vi "Waveform Input.vi"(8 "error in (no error)":errorcluster, 11 "Node Ptr":T1 format="%.0x") -> (0 "error out":errorcluster)   [LabVIEW 2019, in "FPGA Addon System Explorer.lvlib"]
uses:
  FPGA Addon System Explorer.lvlib
  <vilib>/NI VeriStand/Custom Device API/Custom Device Item Ref.ctl
  <vilib>/NI VeriStand/Custom Device API/Custom Device API.lvlib
panel:
  out "Original Name":string
  in  "Units":string
  in  "Header":cluster{"Section Name":string}={"Section Name"="Waveform Input Settings"}
  in  "Description":string
  in  "Name":string
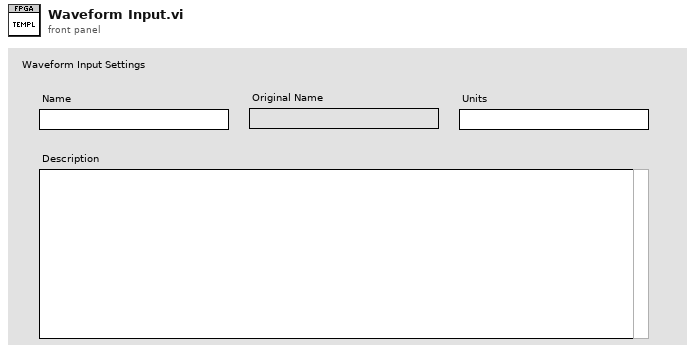
[diagram p1: front panel]
types:
  T1 = typedef "Custom Device API.lvlib/Custom Device Item Ref.ctl" = u64
  T2 = typedef "Custom Device API.lvlib/Custom Device Item Info.ctl" = cluster{"Name":string, "Is Channel":bool, "GUID":string, "Is Waveform":bool}
  T3 = typedef "Custom Device API.lvlib/Custom Device Waveform.ctl" = cluster{"Data Type":T4, "Units":string}
  T4 = typedef "Custom Device API.lvlib/Custom Device Waveform DataType.ctl" = enum16{"Double", "Complex Double"}
  T5 = typedef "Custom Device API.lvlib/Custom Device Commands.ctl" = enum16{"Default", "Item renamed", "Shutdown", "Dynamic button pressed"}
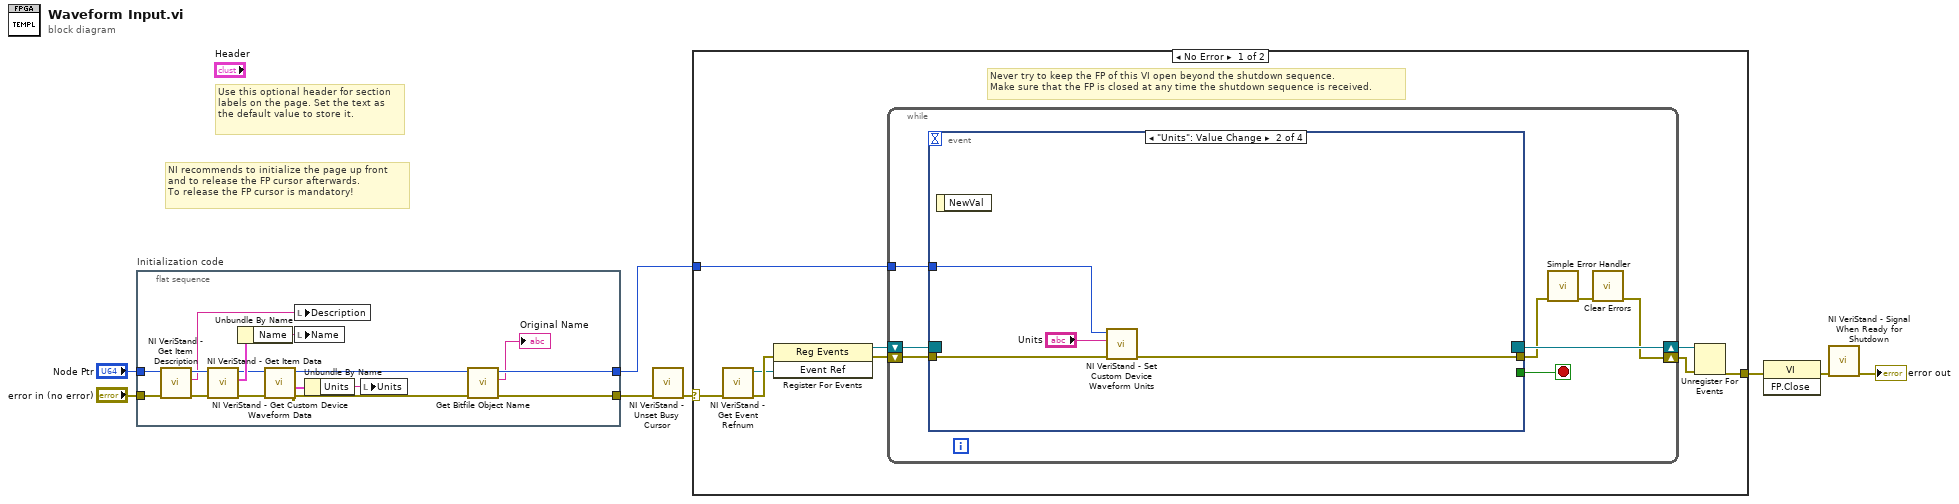
[diagram p0: block diagram]
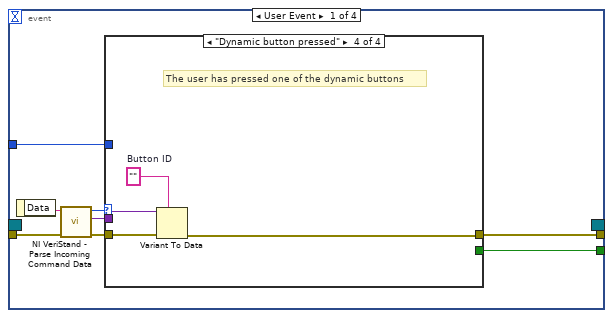
[diagram p2: hidden frame]
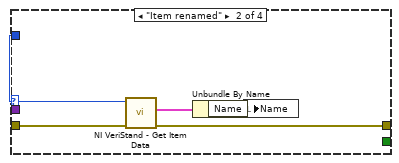
[diagram p4: hidden frame]
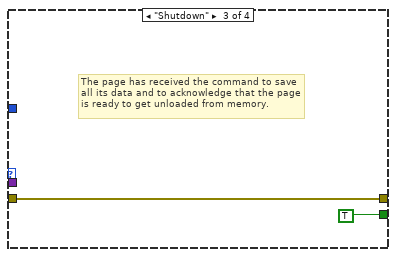
[diagram p5: hidden frame]
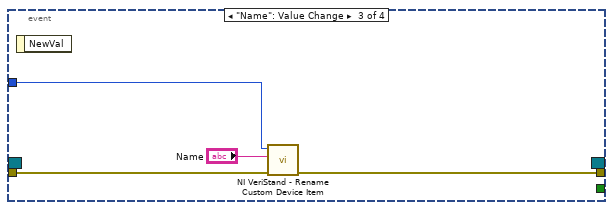
[diagram p6: hidden frame]
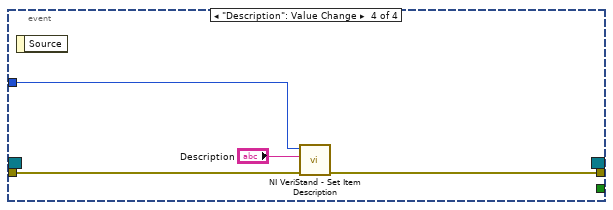
[diagram p7: hidden frame]
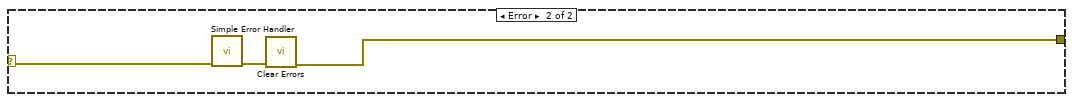
[diagram p8: hidden frame]
diagram:
  # "Use this optional header for section labels on the page. Set the text as the default value to store it."
  # "NI recommends to initialize the page up front\nand to release the FP cursor afterwards.\nTo release the FP cursor is mandatory!"
  n1 = flat-sequence "Initialization code" {
    tunnel: "error in (no error)" -> [w23]
    tunnel: "Node Ptr" -> [w22]
    tunnel: [w13] -> w4
    tunnel: [w10] -> w1
    frame #0 {
      n2 = call <vilib>:"NI VeriStand - Get Item Description.vi"("error in (no error)"=w23, "Item Ref in"=w22) -> ("error out"=w20:errorcluster, "Description"=w21:string, "Item Ref out"=w24:T1)  [unwired: 7 out]
      n3 = call <vilib>:"NI VeriStand - Get Item Data.vi"("error in (no error)"=w20, "Item Ref in"=w24) -> ("error out"=w14:errorcluster, "Item Info"=w19:T2, "Item Ref out"=w15:T1)  [unwired: 7 out]
      n4 = Unbundle By Name(w19) -> ("Name"=w18:string)
      n5 = call <vilib>:"NI VeriStand - Get Custom Device Waveform Data.vi"("error in (no error)"=w14, "Waveform Ref in"=w15) -> ("error out"=w12:errorcluster, "Waveform"=w17:T3, "Waveform Ref out"=w11:T1)  [unwired: 4 in, 3 out]
      n6 = local write "Description"(w21) -> ()
      n7 = local write "Name"(w18) -> ()
      n8 = Unbundle By Name(w17) -> ("Units"=w16:string)
      n9 = local write "Units"(w16) -> ()
      n10 = call "Get Bitfile Object Name.vi"("error in (no error)"=w12, "Item Ref in"=w11) -> ("error out"=w13:errorcluster, "Value"=→"Original Name":string, "Item Ref out"=w10:T1)  [unwired: 7 in]
    }
  }
  n11 = call <vilib>:"NI VeriStand - Unset Busy Cursor.vi"("error in (no error)"=w4) -> ("error out"=w3:errorcluster)  [unwired: 10 out]
  n12 = case shown="No Error" w3 {
    selector: w3 -> [w25 w76]
    tunnel: [w30 w74] -> w8
    tunnel: w1 -> [w26 _]
    frame No Error {
      # "Never try to keep the FP of this VI open beyond the shutdown sequence.\nMake sure that the FP is closed at any time the shutdown sequence is received."
      n13 = call <vilib>:"NI VeriStand - Get Event Refnum.vi"("error in (no error)"=w25) -> ("error out"=w33:errorcluster, "Event Ref"=w29:refnum<user-event>)  [unwired: 9 out]
      n14 = register-events(error in=w33, w29) -> (reference out=w27:refnum<event-registration>, error out=w28:errorcluster)  [unwired: 1 in]
      n15 = while {
        tunnel: w26 -> [w37]
        shift-right: [w34] -> w31
        shift-left: w28 -> [w40]
        shift-right: [w41] -> w32
        shift-left: w27 -> [w39]
        stop <- w38 stop-if-true
        n16 = event shown="[1] \"Units\": Value Change" {
          selector: w39 -> [_ _ _ _]
          dyn-events: [_ _ _ _] -> w41
          timeout: _ -> [_ _ _ _]
          tunnel: w40 -> [w49 w64 w69 w72]
          tunnel: [w45 _ _ _] -> w38
          tunnel: [w44 w63 w68 w71] -> w36
          tunnel: w37 -> [w43 w65 w67 w73]
          event User Event {
            n17 = event-data() -> ("Data"=w48:string)  [unwired: 1 out]
            n18 = call <vilib>:"NI VeriStand - Parse Incoming Command Data.vi"("error in (no error)"=w49, "Incoming data"=w48) -> ("error out"=w47:errorcluster, "Outgoing data"=w42:variant, "Action"=w46:T5)  [unwired: 7 out]
            n19 = case shown="\"Dynamic button pressed\"" w46 {
              tunnel: w47 -> [w50 w55 w56 w61]
              tunnel: [_ _ TRUE _] -> w45
              tunnel: [w50 w52 w56 w58] -> w44
              tunnel: w43 -> [_ w54 _ _]
              tunnel: w42 -> [_ _ _ w60]
              frame "Default", Default {
              }
              frame "Item renamed" {
                n20 = call <vilib>:"NI VeriStand - Get Item Data.vi"("error in (no error)"=w55, "Item Ref in"=w54) -> ("error out"=w52:errorcluster, "Item Info"=w53:T2)  [unwired: 8 out]
                n21 = Unbundle By Name(w53) -> ("Name"=w51:string)
                n22 = local write "Name"(w51) -> ()
              }
              frame "Shutdown" {
                # "The page has received the command to save all its data and to acknowledge that the page is ready to get unloaded from memory."
              }
              frame "Dynamic button pressed" {
                w59 = ""  # Button ID
                # "The user has pressed one of the dynamic buttons"
                n23 = Variant To Data(error in=w61, type=w59, Variant=w60) -> (error out=w58:errorcluster)  [unwired: 1 out]
              }
            }
          }
          event "Units": Value Change {
            n24 = event-data() -> ()  [unwired: 2 out]
            n25 = call <vilib>:"NI VeriStand - Set Custom Device Waveform Units.vi"("error in (no error)"=w64, "Units"="Units", "Waveform Ref in"=w65) -> ("error out"=w63:errorcluster)  [unwired: 7 in, 1 out]
          }
          event "Name": Value Change {
            n26 = event-data() -> ()  [unwired: 2 out]
            n27 = call <vilib>:"NI VeriStand - Rename Custom Device Item.vi"("error in (no error)"=w69, "New Name"="Name", "Item Ref in"=w67) -> ("error out"=w68:errorcluster)  [unwired: 1 in, 7 out]
          }
          event "Description": Value Change {
            n28 = event-data() -> ()  [unwired: 2 out]
            n29 = call <vilib>:"NI VeriStand - Set Item Description.vi"("error in (no error)"=w72, "Description"="Description", "Item Ref in"=w73) -> ("error out"=w71:errorcluster)  [unwired: 8 out]
          }
        }
        n30 = call <vilib>:"Simple Error Handler.vi"("error in (no error)"=w36) -> ("error out"=w35:errorcluster)  [unwired: 1 in, 7 out]
        n31 = call <vilib>:"Clear Errors.vi"("error in (no error)"=w35) -> ("error out"=w34:errorcluster)  [unwired: 1 in, 5 out]
      }
      n32 = Unregister For Events(event registration refnum=w32, error in=w31) -> (error out=w30:errorcluster)
    }
    frame Error {
      n33 = call <vilib>:"Simple Error Handler.vi"("error in (no error)"=w76) -> ("error out"=w75:errorcluster)  [unwired: 1 in, 7 out]
      n34 = call <vilib>:"Clear Errors.vi"("error in (no error)"=w75) -> ("error out"=w74:errorcluster)  [unwired: 1 in, 5 out]
    }
  }
  n35 = invoke class="VI" method="FP.Close"(error in=w8) -> (error out=w7:errorcluster)  [unwired: 2 in, 2 out]
  n36 = call <vilib>:"NI VeriStand - Signal When Ready for Shutdown.vi"("error in (no error)"=w7) -> ("error out"=→"error out":errorcluster)  [unwired: 10 out]
